vi "Test Perform Action.vi"(11 "Test Case In":refnum<class "NI9375 DI Cont CFG.lvclass">) -> (0 "error out":errorcluster, 3 "Test Case Out":refnum<class "NI9375 DI Cont CFG.lvclass">)   [LabVIEW 2024, in "NI9375 DI Cont CFG.lvclass"]
uses:
  NI9375 DI Cont CFG.lvclass
  HAL/Devices/DAQmx/DIO/DI DAQmx Cont CFG/DI DAQmx Cont CFG.lvclass
  HAL/Helper/Digital Waveform Chart/Digital Waveform Chart.lvclass
  <vilib>/Astemes/LUnit/Test Case.lvclass/Test Case.ctl
  7f5aa1ed-7e4e-4c06-b312-a0742ed14d1d.vi
  <vilib>/Astemes/LUnit/Append Pass Result.vi
  <vilib>/Astemes/LUnit/Append Fail Result.vi
  <vilib>/Astemes/LUnit/Run In UI.vi
  <vilib>/Utility/error.llb/Clear Errors.vi
  <vilib>/Waveform/DWDTOps.llb/DWDT Digital to Binary U8.vi
  NI9375 DI Cont CFG.lvclass/NI9375 DI Cont CFG.ctl
  <vilib>/Astemes/LUnit/Test Case.lvclass
  HAL/Configurations/CFG Base/CFG Base.lvclass
  <userlib>/_OpenG.lib/lvdata/lvdata.llb/openg_variant.lvlib
  D:/git/HAL/HAL/Devices/DAQmx/DAQmx Base CFG/DAQmx Base CFG.lvclass
  D:/git/HAL/HAL/Configurations/CFG Base/CFG Base.lvclass
  D:/git/HAL/HAL/Devices/DAQmx/DIO/DI DAQmx Cont CFG/DI DAQmx Cont CFG.lvclass
  C:/Program Files/National Instruments/LabVIEW 2024/vi.lib/Astemes/LUnit/Test Case.lvclass
  C:/Program Files/National Instruments/LabVIEW 2024/vi.lib/Astemes/LUnit/LUnit Runnable.lvclass
  D:/git/HAL/Tests/NI9375 DI Cont CFG/NI9375 DI Cont CFG.lvclass
panel:
  out "Waveform Chart":waveform(dbl)[](graph)
  out "Digital Waveform out":digitalwaveform(waveform)={"t0"=timestamp(0 s since 1904-01-01), "dt"=1.0, "Y"={"transitions"=[], "data"=[]}}
  out "Numeric":i32
  out "Digital Waveform Graph":digitalwaveform(graph)
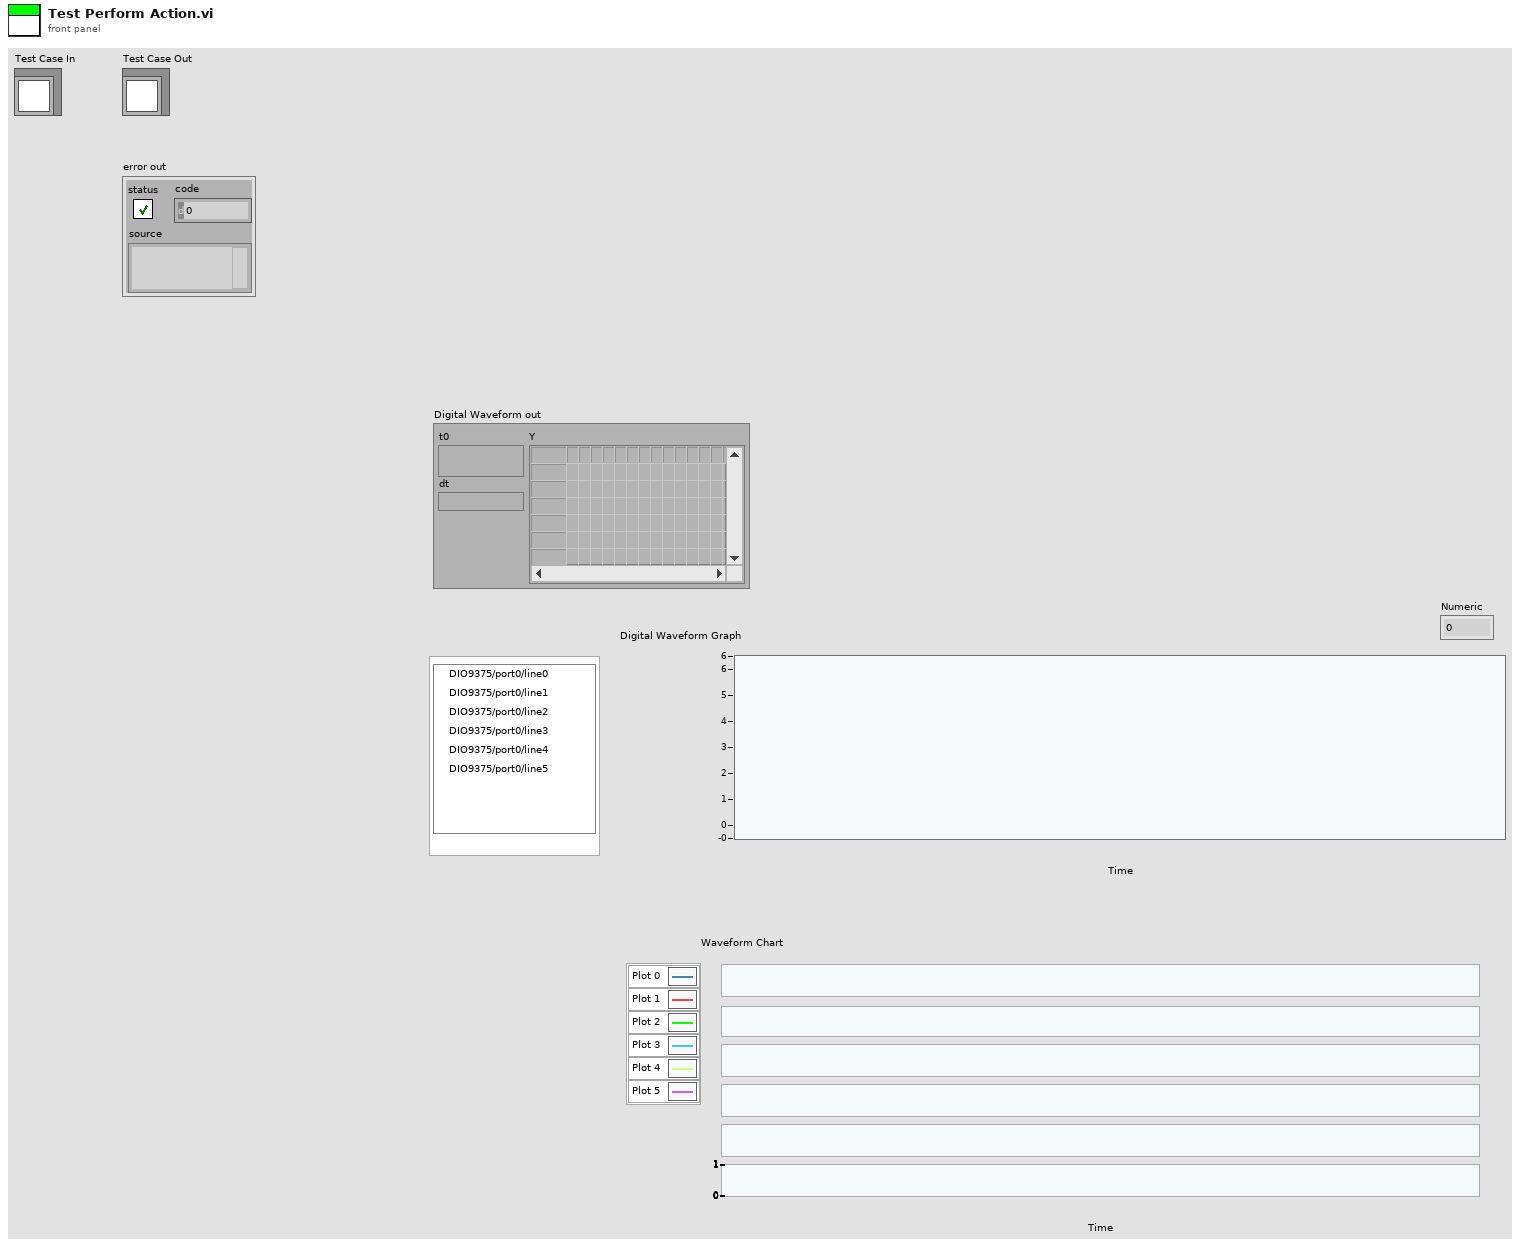
[diagram p1: front panel]
types:
  T1 = typedef "openg_variant.lvlib/Type Descriptor Enumeration__ogtk.ctl" = enum8{"<Null>", "I8", "I16", "I32", "I64", "U8", "U16", "U32", "U64", "SGL", "DBL", "EXT", "CSG", "CDB", "CXT", "0x0F", "0x10", "0x11", "0x12", "0x13", "0x14", "Enum U8", "Enum U16", "Enum U32", "Enum U64", "SGL PQ", "DBL PQ", "EXT PQ", "CSG PQ", "CDB PQ", "CXT PQ", "0x1F", "0x20", "Boolean", "0x22", "0x23", "0x24", "0x25", "0x26", "0x27", "0x28", "0x29", "0x2A", "0x2B", "0x2C", "0x2D", "0x2E", "0x2F", "String", "0x31", "Path", "Pict", "0x34", "0x35", "0x36", "DAQ", "0x38", "0x39", "0x3A", "0x3B", "0x3C", "0x3D", "0x3E", "0x3F", "Array", "0x41", "0x42", "0x43", "0x44", "0x45", "0x46", "0x47", "0x48", "0x49", "0x4A", "0x4B", "0x4C", "0x4D", "0x4E", "0x4F", "Cluster", "0x51", "0x52", "Variant", "Waveform", "0x55", "0x56", "0x57", "0x58", "0x59", "0x5A", "0x5B", "0x5C", "0x5D", "0x5E", "Fixed Point", "0x60", "0x61", "0x62", "0x63", "0x64", "0x65", "0x66", "0x67", "0x68", "0x69", "0x6A", "0x6B", "0x6C", "0x6D", "0x6E", "0x6F", "Refnum", "0x71", "0x72", "Set Collection", "Map Collection"}
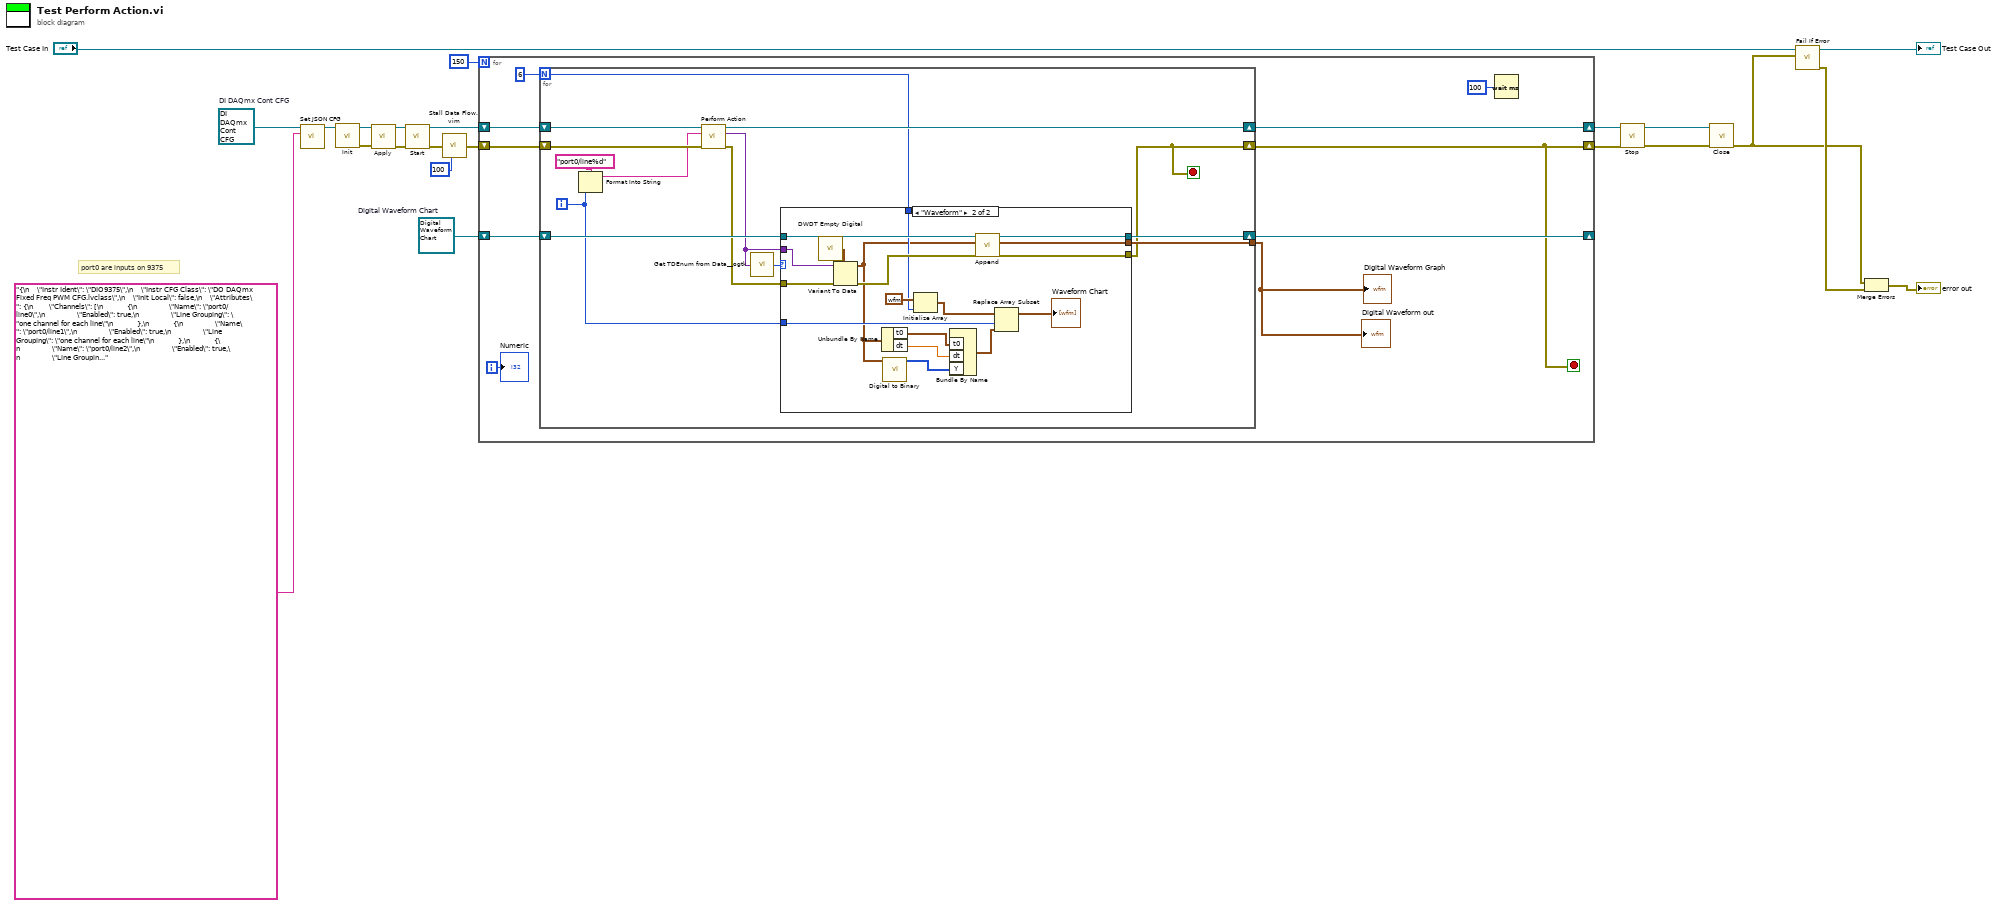
[diagram p0: block diagram]
diagram:
  w1 = refnum<class "Digital Waveform Chart.lvclass"> refnum  # Digital Waveform Chart
  w8 = refnum<class "DI DAQmx Cont CFG.lvclass"> refnum  # DI DAQmx Cont CFG
  # "port0 are inputs on 9375"
  n1 = call "Set JSON CFG.vi"("<JSON>CFG"="{\n    \"Instr Ident\": \"DIO9375\",\n    \"Instr CFG Class\": \"DO DAQmx Fixed Freq PWM CFG.lvclass\",\n    \"Init Local\": false,\n    \"Attributes\": {\n        \"Channels\": [\n            {\n                \"Name\": \"port0/line0\",\n                \"Enabled\": true,\n                \"Line Grouping\": \"one channel for each line\"\n            },\n            {\n                \"Name\": \"port0/line1\",\n                \"Enabled\": true,\n                \"Line Grouping\": \"one channel for each line\"\n            },\n            {\n                \"Name\": \"port0/line2\",\n                \"Enabled\": true,\n                \"Line Grouping\": \"one channel for each line\"\n            },\n            {\n                \"Name\": \"port0/line3\",\n                \"Enabled\": true,\n                \"Line Grouping\": \"one channel for each line\"\n            },\n            {\n                \"Name\": \"port0/line4\",\n                \"Enabled\": true,\n                \"Line Grouping\": \"one channel for each line\"\n            },\n            {\n                \"Name\": \"port0/line5\",\n                \"Enabled\": true,\n                \"Line Grouping\": \"one channel for each line\"\n            }\n        ],\n        \"Timing\": {\n            \"Type\": \"Sample Clock\",\n            \"Samples per Channel\": 100,\n            \"Sample Mode\": \"Continuous Samples\",\n            \"Sample Rate\": 11,\n            \"Sample Clock Source\": \"OnboardClock\",\n            \"Active Edge\": \"Rising\"\n        },\n        \"Trigger\": {\n            \"Trigger Type\": \"No Trigger\"\n        },\n        \"Generation\": {\n            \"Regen Mode\": \"Allow Regeneration\"\n        }\n    }\n}" ("<JSON> CFG"), "CFG Base in"=w8) -> ("CFG Base out"=w11:refnum<class "DI DAQmx Cont CFG.lvclass">)  [unwired: 9 in]
  n2 = call-dynamic "Init.vi"("DAQmx Base CFG in"=w11) -> ("error out"=w19:errorcluster, "DAQmx Base CFG out"=w10:refnum<class "DI DAQmx Cont CFG.lvclass">)  [unwired: 9 in]
  n3 = call-dynamic "Apply.vi"("error in"=w19, "DAQmx Base CFG in"=w10) -> ("error out"=w18:errorcluster, "DAQmx Base CFG out"=w17:refnum<class "DI DAQmx Cont CFG.lvclass">)  [unwired: 8 in]
  n4 = call-dynamic "Start.vi"("error in"=w18, "DAQmx Base CFG in"=w17) -> ("error out"=w2:errorcluster, "DAQmx Base CFG out"=w16:refnum<class "DI DAQmx Cont CFG.lvclass">)  [unwired: 8 in]
  n5 = call "Stall Data Flow.vim"("value in"=w2, "milliseconds to wait"=u32 100) -> ("value out"=w3:errorcluster)  [unwired: 1 out]
  n6 = for {
    N: 150 -> [_]
    shift-right: [w30] -> w15
    shift-left: w16 -> [w31]
    shift-right: [w26] -> w14
    shift-left: w3 -> [w25]
    shift-right: [w28] -> _
    shift-left: w1 -> [w29]
    i -> [w27]
    stop <- w26 stop-if-true
    n7 = for {
      N: 6 -> [w34]
      shift-right: [w36] -> w26
      shift-left: w25 -> [w45]
      shift-right: [w44] -> w30
      shift-left: w31 -> [w46]
      shift-right: [w39] -> w28
      shift-left: w29 -> [w40]
      tunnel: [w38] -> w23
      i -> [w33]
      stop <- w36 stop-if-true
      n8 = Format Into String(format string="port0/line%d", w33) -> (resulting string=w42:string)  [unwired: 2 in, 1 out]
      n9 = call-dynamic "Perform Action.vi"("error in"=w45, "Input"=w42, "DI DAQmx Cont CFG in"=w46) -> ("error out"=w37:errorcluster, "Output"=w35:variant, "DI DAQmx Cont CFG out"=w44:refnum<class "DI DAQmx Cont CFG.lvclass">)  [unwired: 6 in]
      n10 = call <userlib>:"Get TDEnum from Data__ogtk.vi"("Data"=w35) -> ("Type Descriptor Enumeration"=w41:T1)  [unwired: 4 in]
      n11 = case shown="\"Waveform\"" w41 {
        tunnel: w35 -> [_ w65]
        tunnel: w40 -> [w48 w64]
        tunnel: [w48 w63] -> w39
        tunnel: [_ w61] -> w38
        tunnel: [w47 w60] -> w36
        tunnel: w37 -> [w47 w59]
        tunnel: w34 -> [_ w57]
        tunnel: w33 -> [_ w54]
        frame Default {
        }
        frame "Waveform" {
          n12 = call <vilib>:"DWDT Empty Digital.vi"() -> ("digital waveform out"=w66:digitalwaveform)  [unwired: 5 in]
          n13 = Variant To Data(error in=w59, type=w66, Variant=w65) -> (data=w53:digitalwaveform, error out=w62:errorcluster)
          n14 = Unbundle By Name(w53) -> ("t0"=w51:timestamp, "dt"=w50:dbl)
          n15 = call-poly <vilib>:"Digital to Binary.vi"("digital waveform"=w53) -> ("binary array"=w49:u8[])  [unwired: 9 in, 1 out]
          n16 = Initialize Array(waveform(dbl) {"t0"=timestamp(0 s since 1904-01-01), "dt"=1.0, "Y"=[]} ("Waveform"), w57) -> (w55:waveform(dbl)[])
          n17 = Bundle By Name("t0"=w51, "dt"=w50, "Y"=w49) -> (w52:waveform(u8))  [unwired: 1 in]
          n18 = call "Append.vi"("error in"=w62, "Digital Waveform in"=w53, "Digital Waveform Chart in"=w64) -> ("error out"=w60:errorcluster, "Digital Waveform out"=w61:digitalwaveform, "Digital Waveform Chart out"=w63:refnum<class "Digital Waveform Chart.lvclass">)  [unwired: 6 in]
          n19 = Replace Array Subset(array=w55, new element=w52, index=w54) -> (→"Waveform Chart":waveform(dbl)[])
        }
      }
    }
    "Digital Waveform Graph" <- w23
    "Digital Waveform out" <- w23
    n20 = Wait (ms)(milliseconds to wait=u32 100) -> ()  [unwired: 1 out]
    "Numeric" <- w27
  }
  n21 = call-dynamic "Stop.vi"("error in"=w14, "DAQmx Base CFG in"=w15) -> ("error out"=w13:errorcluster, "DAQmx Base CFG out"=w12:refnum<class "DI DAQmx Cont CFG.lvclass">)  [unwired: 8 in]
  n22 = call-dynamic "Close.vi"("error in"=w13, "DAQmx Base CFG in"=w12) -> ("error out"=w6:errorcluster)  [unwired: 8 in, 1 out]
  n23 = call <vilib>:"Fail If Error.vi"("Assert error"=w6, "LUnit Test Case In"="Test Case In") -> ("error out"=w20:errorcluster, "LUnit Test Case Out"=→"Test Case Out":refnum<class "NI9375 DI Cont CFG.lvclass">)  [unwired: 8 in]
  n24 = Merge Errors(w6, w20) -> (→"error out":errorcluster)
